vi "getAllTables.vi"(8 "error in (no error)":errorcluster, 11 "xwpfReader in":refnum<class "xwpfReader.lvclass">) -> (0 "error out":errorcluster, 2 "Tables":string[][][](array[string]), 3 "xwpfReader out":refnum<class "xwpfReader.lvclass">)   [LabVIEW 2017, in "LabVIEW NPOI.lvlib" / "xwpfReader.lvclass"]
doc: "Get all the paragraphs."
uses:
  xwpfReader.lvclass
  xwpfReader.lvclass/xwpfReader.ctl
  C:/Users/Neo/Desktop/Dev_Tools_BR/LabVIEW_NPOI/lib/NPOI 2.1.1/NPOI.OOXML.dll
  lib/NPOI 2.1.1/NPOI.OOXML.dll
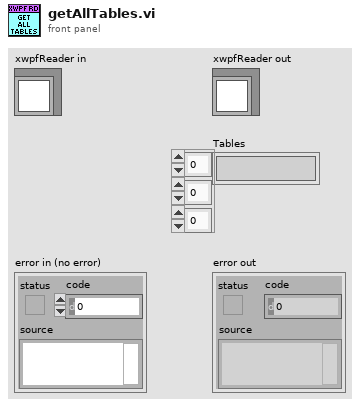
[diagram p1: front panel]
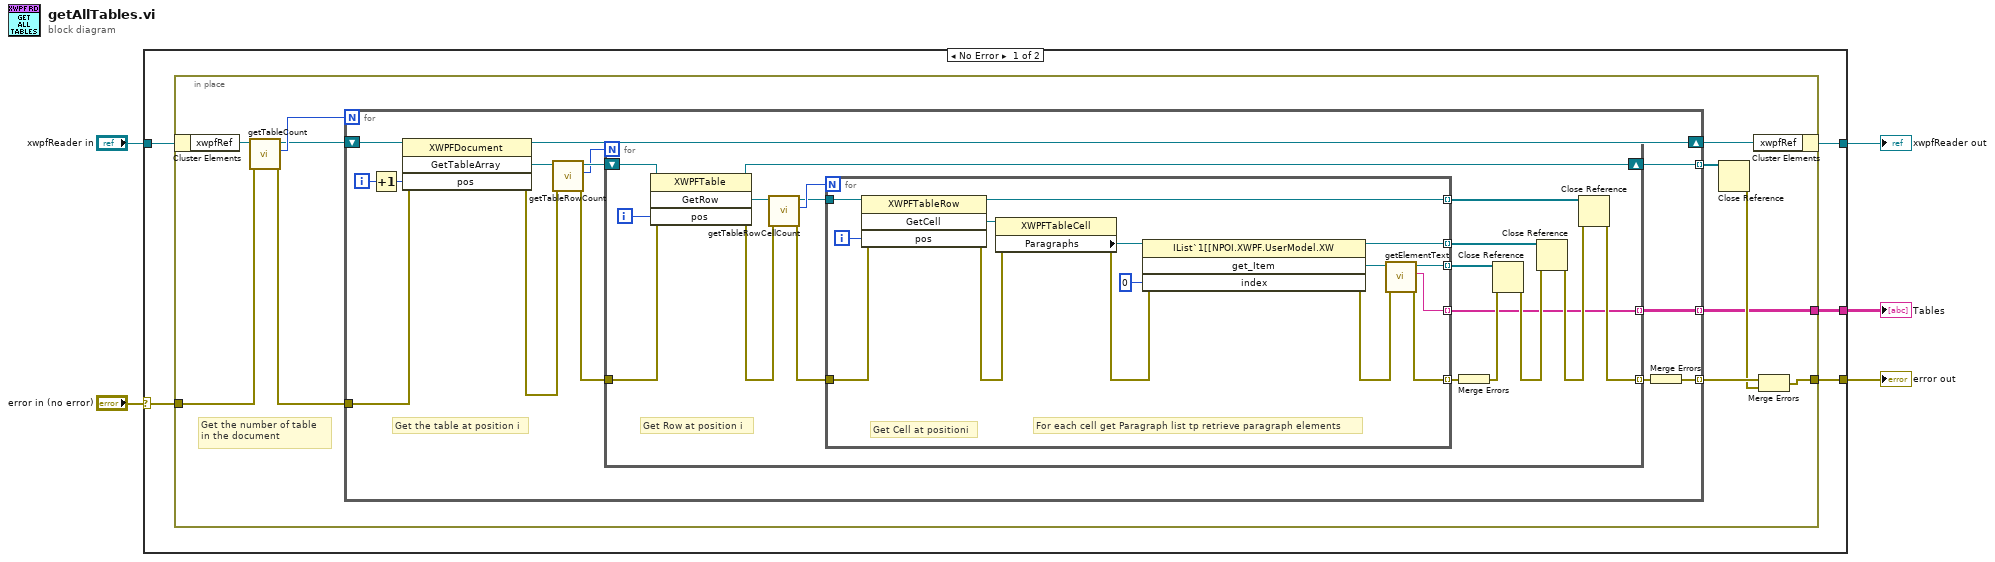
[diagram p0: block diagram]
diagram:
  n1 = case shown="No Error" "error in (no error)" {
    selector: "error in (no error)" -> [w8 w70]
    tunnel: [w7 w70] -> w4
    tunnel: [w10 w69] -> w2
    tunnel: "xwpfReader in" -> [w9 w69]
    tunnel: [w6 _] -> w1
    frame No Error {
      n2 = in-place {
        in-place-border: w8 -> [w19]
        in-place-border: [w15] -> w7
        in-place-border: [w12] -> w6
        # "Get the number of table \nin the document"
        n3 = in-place-cluster #1(w9) -> ("xwpfRef"=w21:refnum<k24>)
        n4 = call "getTableCount.vi"("error in (no error)"=w19, ".NET Refnum in"=w21) -> ("error out"=w11:errorcluster, "Table Count"=w20:i32, ".NET Refnum out"=w17:refnum<k24>)  [unwired: 7 in]
        n5 = for {
          N: w20 -> [_]
          tunnel: w11 -> [w34]
          tunnel: [w22] -> w18 mode=indexing
          shift-right: [w28] -> w13
          shift-left: w17 -> [w29]
          tunnel: [w33] -> w16 mode=indexing
          tunnel: [w31] -> w12 mode=indexing
          i -> [w35]
          # "Get the table at position i"
          n6 = Increment(x=w35) -> (x+1=w30:i32)
          n7 = invoke class="XWPFDocument" method="GetTableArray"(reference=w29, error in=w34, "pos"=w30) -> (reference out=w28:refnum<k24>, error out=w24:errorcluster, "GetTableArray"=w27:refnum<k24>)  [unwired: 1 in, 1 out]
          n8 = call "getTableRowCount.vi"("error in (no error)"=w24, "Table"=w27) -> ("error out"=w23:errorcluster, "Count"=w25:i32, "Table"=w26:refnum<k24>)  [unwired: 7 in]
          n9 = for {
            N: w25 -> [_]
            tunnel: w23 -> [w52]
            tunnel: [w37] -> w32 mode=indexing
            tunnel: [w36] -> w31 mode=indexing
            shift-right: [w51] -> w33
            shift-left: w26 -> [w53]
            i -> [w49]
            # "Get Row at position i"
            n10 = invoke class="XWPFTable" method="GetRow"(reference=w53, error in=w52, "pos"=w49) -> (reference out=w51:refnum<k24>, error out=w45:errorcluster, "GetRow"=w48:refnum<k24>)  [unwired: 1 in, 1 out]
            n11 = call "getTableRowCellCount.vi"("error in (no error)"=w45, "TableRow in"=w48) -> ("error out"=w44:errorcluster, "Count"=w47:i32, "TableRow out"=w46:refnum<k24>)  [unwired: 7 in]
            n12 = for {
              N: w47 -> [_]
              tunnel: w46 -> [w68]
              tunnel: [w67] -> w50 mode=indexing
              tunnel: w44 -> [w66]
              tunnel: [w60] -> w36 mode=indexing
              tunnel: [w56] -> w43 mode=indexing
              tunnel: [w55] -> w42 mode=indexing
              tunnel: [w54] -> w40 mode=indexing
              i -> [w65]
              # "For each cell get Paragraph list tp retrieve paragraph elements"
              # "Get Cell at positioni"
              n13 = invoke class="XWPFTableRow" method="GetCell"(reference=w68, error in=w66, "pos"=w65) -> (reference out=w67:refnum<k24>, error out=w57:errorcluster, "GetCell"=w64:refnum<k24>)  [unwired: 1 in, 1 out]
              n14 = property class="XWPFTableCell"(reference=w64, error in=w57) -> (error out=w58:errorcluster, "Paragraphs"=w62:refnum<k24>)  [unwired: 1 out]
              n15 = invoke class="IList`1[[NPOI.XWPF.UserModel.XW" method="get_Item"(reference=w62, error in=w58, "index"=0) -> (reference out=w54:refnum<k24>, error out=w59:errorcluster, "get_Item"=w61:refnum<k24>)  [unwired: 1 in, 1 out]
              n16 = call "getElementText.vi"("error in (no error)"=w59, "Paragraph in"=w61) -> ("error out"=w55:errorcluster, "Text"=w60:string, "Paragraph out"=w56:refnum<k24>)  [unwired: 7 in]
            }
            n17 = Merge Errors(w42) -> (w41:errorcluster)
            n18 = Close Reference(reference=w43, error in (no error)=w41) -> (error out=w38:errorcluster)
            n19 = Close Reference(reference=w40, error in (no error)=w38) -> (error out=w39:errorcluster)
            n20 = Close Reference(reference=w50, error in (no error)=w39) -> (error out=w37:errorcluster)
          }
          n21 = Merge Errors(w32) -> (w22:errorcluster)
        }
        n22 = Close Reference(reference=w16) -> (error out=w14:errorcluster)  [unwired: 1 in]
        n23 = in-place-cluster #1("xwpfRef"=w13) -> (w10:refnum<class "xwpfReader.lvclass">)
        n24 = Merge Errors(w18, w14) -> (w15:errorcluster)
      }
    }
    frame Error {
    }
  }
  "error out" <- w4
  "xwpfReader out" <- w2
  "Tables" <- w1
